vi "WindowLock.vi"() -> ()   [LabVIEW 2017]
uses:
  <vilib>/DAQmx/read.llb/DAQmx Read (Analog 1D DBL NChan 1Samp).vi
  <vilib>/DAQmx/create/channels.llb/DAQmx Create Channel (AI-Current-Basic).vi
  <vilib>/DAQmx/configure/timing.llb/DAQmx Timing (Sample Clock).vi
  <vilib>/DAQmx/miscellaneous.llb/DAQmx Fill In Error Info.vi
panel:
  out "SamplingRate":i32
  out "DISTANCE":string
  out "FORCE":string
  out "NumDistance":dbl
  out "NumForce":dbl
  in  "stop":bool
  out "error out":errorcluster
  # "/Sec."
  # "SAMPLING RATE"
  # "WDW LOCK"
  # "WDW LOCK"
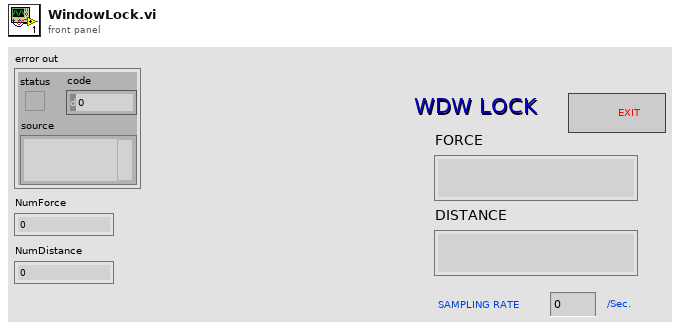
[diagram p1: front panel]
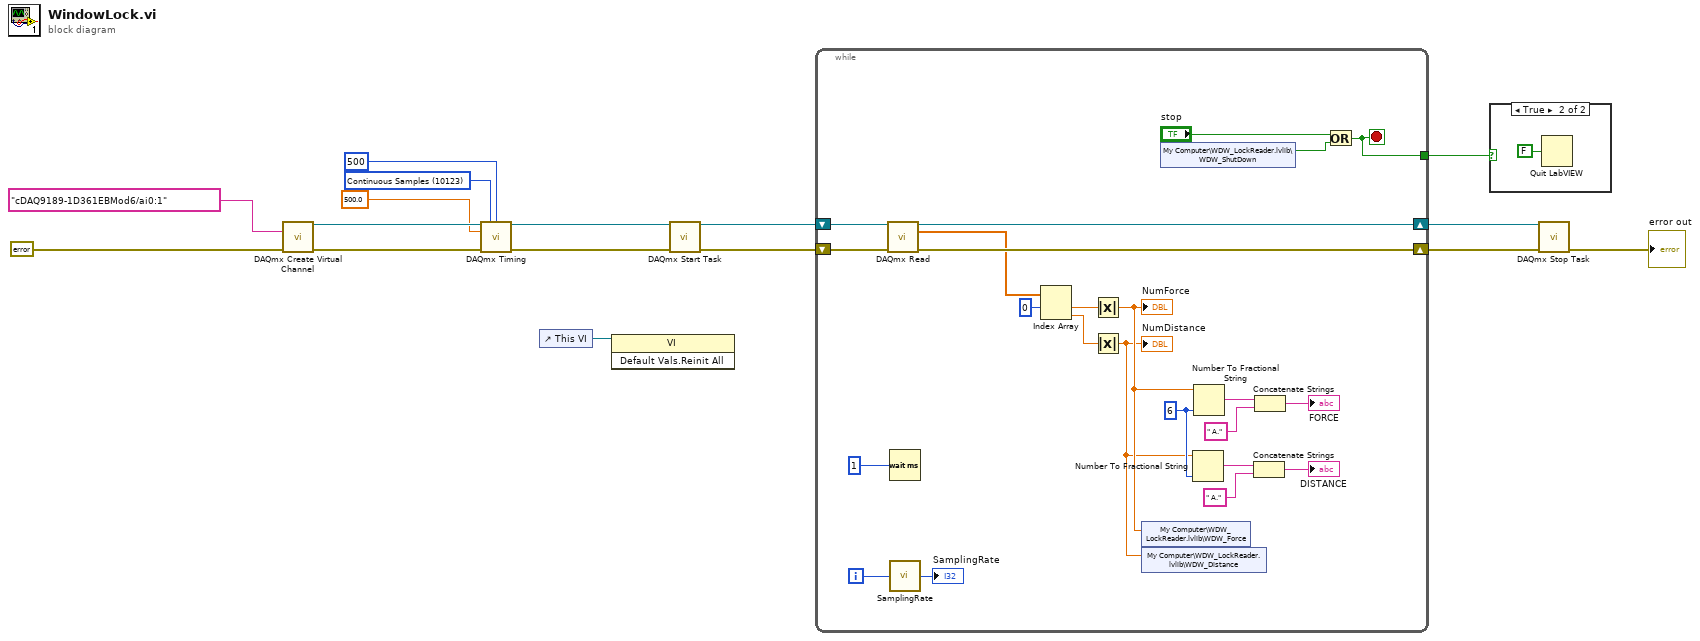
[diagram p0: block diagram]
diagram:
  w2 = 10123 items=["Finite Samples"=10178, "Continuous Samples"=10123, "Hardware Timed Single Point"=12522] ("sample mode")
  n1 = call-poly <vilib>:"DAQmx Create Virtual Channel.vi"("physical channels"=tag "cDAQ9189-1D361EBMod6/ai0:1", "error in"=errorcluster {"status"=FALSE, "code"=0, "source"=""} ("error constant")) -> ("task out"=w7:refnum<k21>, "error out"=w6:errorcluster)  [unwired: 12 in]
  n2 = call-poly <vilib>:"DAQmx Timing.vi"("task/channels in"=w7, "sample mode"=w2, "samples per channel"=500, "rate"=500.0, "error in"=w6) -> ("task out"=w4:refnum<k21>, "error out"=w5:errorcluster)  [unwired: 9 in]
  n3 = control-ref of="This VI"() -> (w9:refnum<vi>)
  n4 = invoke class="VI" method="Default Vals.Reinit All"(reference=w9) -> ()  [unwired: 2 in, 3 out]
  n5 = call <vilib>:"DAQmx Start Task.vi"("task/channels in"=w4, "error in"=w5) -> ("task out"=w15:refnum<k21>, "error out"=w14:errorcluster)  [unwired: 12 in]
  n6 = while {
    shift-right: [w37] -> w12
    shift-left: w15 -> [w39]
    shift-right: [w36] -> w11
    shift-left: w14 -> [w38]
    tunnel: [w20] -> w8
    i -> [w24]
    stop <- w20 stop-if-true
    w31 = i16 6 ("precision (6)")
    n7 = call-poly <vilib>:"DAQmx Read.vi"("task/channels in"=w39, "error in"=w38) -> ("task out"=w37:refnum<k21>, "data"=w34:dbl[], "error out"=w36:errorcluster)  [unwired: 11 in]
    n8 = Wait (ms)(milliseconds to wait=u32 1) -> ()  [unwired: 1 out]
    n9 = call "SamplingRate.vi"("Loop In"=w24) -> ("SamplingRate"=→"SamplingRate":i32)  [unwired: 4 in]
    n10 = Index Array(array=w34, index #1=0 ("index")) -> (element #1=w35:dbl, element #2=w32:dbl)  [unwired: 1 in]
    n11 = Absolute Value(x=w35) -> (abs(x)=w22:dbl)
    "NumForce" <- w22
    n12 = Absolute Value(x=w32) -> (abs(x)=w21:dbl)
    "NumDistance" <- w21
    n13 = shared-variable "My Computer\\WDW_LockReader.lvlib\\WDW_Force"(w22) -> ()  [unwired: 1 in, 1 out]
    n14 = shared-variable "My Computer\\WDW_LockReader.lvlib\\WDW_Distance"(w21) -> ()  [unwired: 1 in, 1 out]
    n15 = shared-variable "My Computer\\WDW_LockReader.lvlib\\WDW_ShutDown"() -> (w18:bool)  [unwired: 1 in, 1 out]
    n16 = Number To Fractional String(number=w21, precision (6)=w31) -> (F-format string=w29:string)  [unwired: 2 in]
    n17 = Number To Fractional String(number=w22, precision (6)=w31) -> (F-format string=w25:string)  [unwired: 2 in]
    n18 = Concatenate Strings(w29, " A." ("string")) -> (→"DISTANCE":string)
    n19 = Concatenate Strings(w25, " A." ("string")) -> (→"FORCE":string)
    n20 = Or(x="stop", y=w18) -> (x .or. y?=w20:bool)
  }
  n21 = case shown="True" w8 {
    frame False {
    }
    frame True {
      n22 = Quit LabVIEW(quit? (T)=FALSE) -> ()
    }
  }
  n23 = call <vilib>:"DAQmx Stop Task.vi"("task/channels in"=w12, "error in"=w11) -> ("error out"=→"error out":errorcluster)  [unwired: 12 in, 1 out]
